vi "String to 1D Array.vi"(5 "ignore duplicate delimiters? (F=No)":bool, 7 "delimiter (Tab)":string="\t", 10 "String":string) -> (1 "Array of Strings":string[](array[string]))   [LabVIEW 2020]
doc: "Converts delimited string to a 1D array."
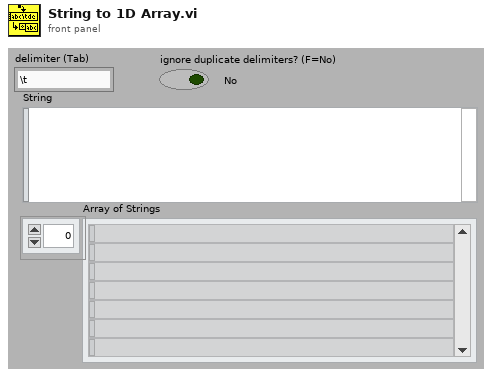
[diagram p1: front panel]
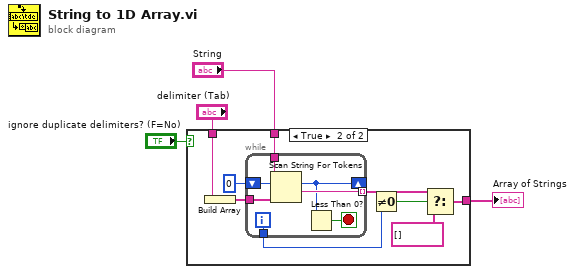
[diagram p0: block diagram]
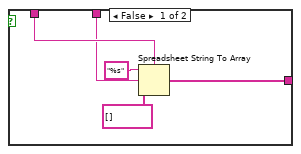
[diagram p2: hidden frame]
diagram:
  n1 = case shown="True" "ignore duplicate delimiters? (F=No)" {
    tunnel: [w7 w11] -> w2
    tunnel: "delimiter (Tab)" -> [w6 w12]
    tunnel: "String" -> [w5 w10]
    frame False {
      n2 = Spreadsheet String To Array(delimiter (Tab)=w6, format string="%s", spreadsheet string=w5, array type (2D Dbl)=string[] [] ("Array Constant")) -> (array=w7:string[])
    }
    frame True {
      n3 = Build Array(w12) -> (w17:string[])
      n4 = while {
        shift-right: [w23] -> _
        shift-left: 0 ("offset past token") -> [w25]
        tunnel: [w24] -> w16 mode=indexing
        tunnel: w10 -> [w21]
        tunnel: w17 -> [w20]
        tunnel: [w19] -> w15
        i -> [w19]
        stop <- w22 stop-if-true
        n5 = Scan String For Tokens(6:w20, 8:w25, 9:w21) -> (1:w24:string, 2:w23:i32)  [unwired: 3 in, 2 out]
        n6 = Less Than 0?(x=w23) -> (x < 0?=w22:bool)
      }
      n7 = Not Equal To 0?(x=w15) -> (x != 0?=w14:bool)
      n8 = Select(t=w16, s=w14, f=string[] []) -> (s? t:f=w11:string[])
    }
  }
  "Array of Strings" <- w2
